vi "Get Plugin UIs.vi"(8 "error in (no error)":errorcluster, 11 "Component UI in":refnum<class "Component User Interfaces.lvclass">) -> (0 "error out":errorcluster, 2 "Plugin Settings UI":refnum<class "User Interface.lvclass">, 3 "Component UI out":refnum<class "Component User Interfaces.lvclass">)   [LabVIEW 2017, in "DSF Core.lvlib" / "Component User Interfaces.lvclass"]
uses:
  Component User Interfaces.lvclass
  User Interface/User Interface.lvclass
  Component User Interfaces.lvclass/Component User Interfaces.ctl
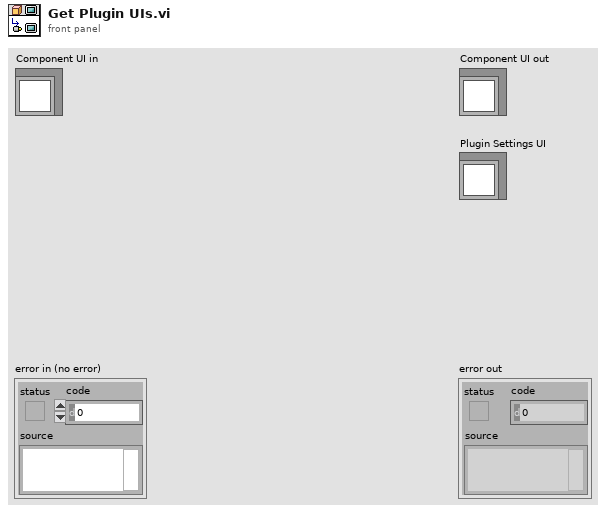
[diagram p1: front panel]
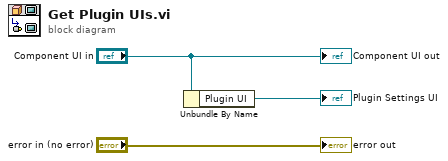
[diagram p0: block diagram]
diagram:
  n1 = Unbundle By Name("Component UI in") -> ("Plugin UI"=→"Plugin Settings UI":refnum<class "User Interface.lvclass">)
  "error out" <- "error in (no error)"
  "Component UI out" <- "Component UI in"
